vi "电阻单次采集.vi"(8 "错误输入（无错误）":errorcluster, 10 "通道数":i32, 11 "VISA引用句柄输入":refnum<visa-resource-name>) -> (0 "错误输出":errorcluster, 2 "测量结果":dbl, 3 "VISA引用句柄输出":refnum<visa-resource-name>, 5 "Scan List (Empty: front panel)":string)   [LabVIEW 2015]
uses:
  Keithley 27XX/Public/Configure/Data/Read Single Point.vi
  Keithley 27XX/Keithley 27XX.lvlib
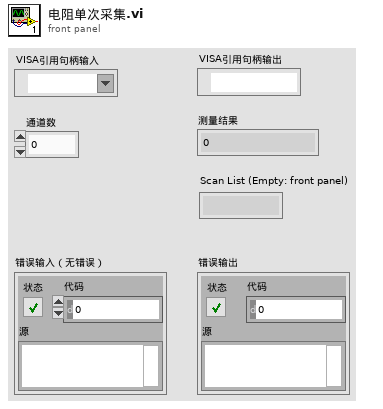
[diagram p1: front panel]
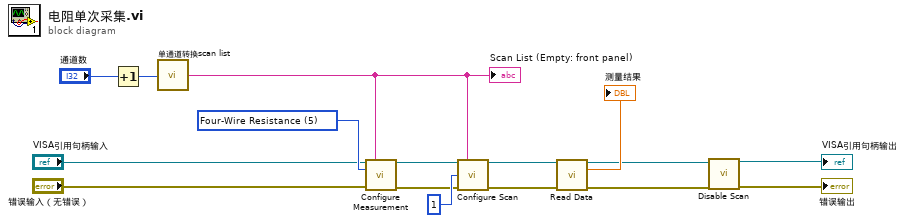
[diagram p0: block diagram]
diagram:
  w9 = u16 5 items=["DC Voltage", "AC Voltage", "DC Current", "AC Current", "Resistance", "Four-Wire Resistance", "Temperature (C)", "Frequency", "Period", "Continuity"] ("Function (0: DC Voltage)")
  n1 = Increment(x="通道数") -> (x+1=w1:i32)
  n2 = call "单通道转换scan list.vi"("测量通道数"=w1) -> ("Scan List"=w10:string)
  "Scan List (Empty: front panel)" <- w10
  n3 = call "Configure Measurement.vi"("VISA resource name"="VISA引用句柄输入", "Scan List (Empty)"=w10, "Function (0: DC Voltage)"=w9, "error in (no error)"="错误输入（无错误）") -> ("VISA resource name out"=w3:refnum<visa-resource-name>, "error out"=w4:errorcluster)  [unwired: 10 in]
  n4 = call "Configure Scan.vi"("VISA resource name"=w3, "Channel List (101:110)"=w10, "Sample Count (100)"=1 ("测量次数"), "error in (no error)"=w4) -> ("VISA resource name out"=w8:refnum<visa-resource-name>, "error out"=w7:errorcluster)  [unwired: 10 in]
  n5 = call-poly "Read Data.vi"("VISA resource name"=w8, "error in (no error)"=w7) -> ("VISA resource name out"=w12:refnum<visa-resource-name>, "Measurement Data"=→"测量结果":dbl, "error out"=w13:errorcluster)  [unwired: 11 in]
  n6 = call "Disable Scan.vi"("VISA resource name"=w12, "error in (no error)"=w13) -> ("VISA resource name out"=→"VISA引用句柄输出":refnum<visa-resource-name>, "error out"=→"错误输出":errorcluster)  [unwired: 12 in]
